vi "Get FPGA Reference.vi"(8 "error in":errorcluster, 11 "Session In":T1) -> (0 "error out":errorcluster, 2 "Ex FPGA Ref":T2, 3 "Session Out":T1)   [LabVIEW 2014, in "Exscalabar FPGA.lvclass"]
doc: "Retrieve the reference to the FPGA session."
uses:
  Exscalabar FPGA.lvclass
  <userlib>/_Session Fwk/Typedefs/Session Handle.ctl
  <userlib>/_Session Fwk/Session - Root.lvclass
  R FPGA Ref.ctl
  Exscalabar FPGA.lvclass/Exscalabar FPGA.ctl
  Read Ex FPGA Ref.vi
  PAS/ePAS Library.lvlib
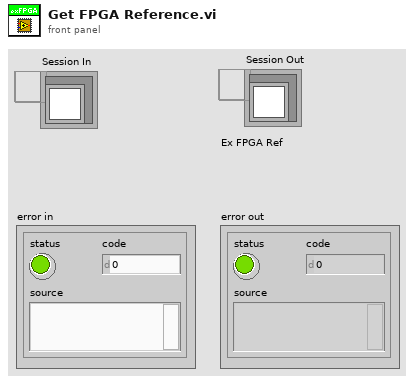
[diagram p1: front panel]
types:
  T1 = typedef "Session - Root.lvclass/Session Handle.ctl" = refnum<data-value>
  T2 = typedef "ePAS Library.lvlib/R FPGA Ref.ctl" = refnum<k20>
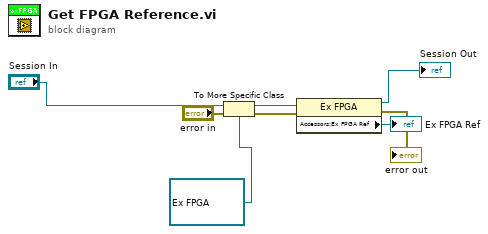
[diagram p0: block diagram]
diagram:
  n1 = To More Specific Class(target class=refnum<data-value> refnum ("Session Handle"), reference="Session In", error in="error in") -> (specific class reference=w6:refnum<data-value>, error out=w5:errorcluster)
  n2 = property class="Ex FPGA"(reference=w6, error in=w5) -> (reference out=→"Session Out":refnum<data-value>, error out=→"error out":errorcluster, "Accessors:Ex FPGA Ref"=→"Ex FPGA Ref":T2)
